vi "MHM ReadSens.vi"(8 "error in (no error)":errorcluster, 11 "ulMHMHandle":u32) -> (0 "error out":errorcluster, 2 "pSensorDataStruct":T1, 3 "function return":u32)   [LabVIEW 2019, in "MHM_1SL_interface.lvlib"]
uses:
  MHM_1SL_interface.lvlib
  lib/MHM_1SL_interface.dll
panel:
  in  "pSensorDataStruct":T1
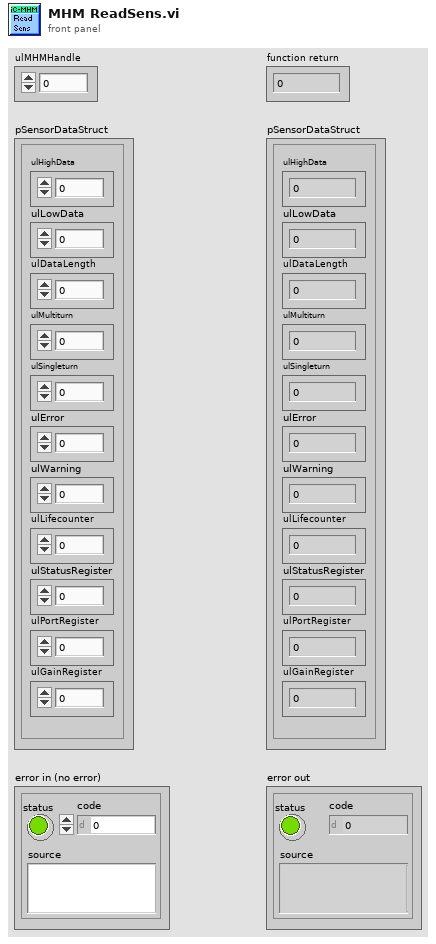
[diagram p1: front panel]
types:
  T1 = cluster{"ulHighData":u32, "ulLowData":u32, "ulDataLength":u32, "ulMultiturn":u32, "ulSingleturn":u32, "ulError":u32, "ulWarning":u32, "ulLifecounter":u32, "ulStatusRegister":u32, "ulPortRegister":u32, "ulGainRegister":u32}
  T2 = cluster{"pulMultiturn":u32, "pulSingleturn":u32, "pulError":u32, "pulWarning":u32, "pulLifecounter":u32, "pulStatusRegister":u32, "pulPortRegister":u32, "pulGainRegister":u32, "pulHighData":u32, "pulLowData":u32, "pulDataLength":u32}
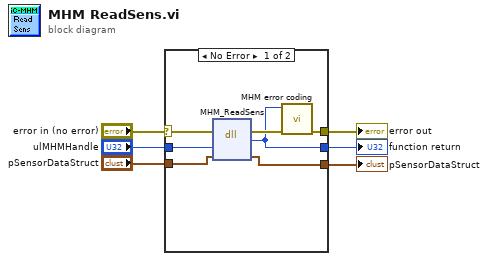
[diagram p0: block diagram]
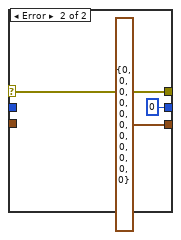
[diagram p2: hidden frame]
diagram:
  n1 = case shown="No Error" "error in (no error)" {
    selector: "error in (no error)" -> [w13 w16]
    tunnel: "ulMHMHandle" -> [w12 _]
    tunnel: [w10 w16] -> w4
    tunnel: [w9 u32 0 ("return type")] -> w3
    tunnel: "pSensorDataStruct" -> [w8 _]
    tunnel: [w7 T2 {"pulMultiturn"=0, "pulSingleturn"=0, "pulError"=0, "pulWarning"=0, "pulLifecounter"=0, "pulStatusRegister"=0, "pulPortRegister"=0, "pulGainRegister"=0, "pulHighData"=0, "pulLowData"=0, "pulDataLength"=0} ("pSensorDataStruct")] -> w1
    frame No Error {
      n2 = dll-call lib="C:/workspace/project/scancon/MHM_1SL_interface_4.4.0/lv_interface/lib/MHM_1SL_interface.dll" fn="MHM_ReadSens"(error in=w13, "ulMHMHandle"=w12, "pSensorDataStruct"=w8) -> (error out=w11:errorcluster, "return type"=w9:u32, "pSensorDataStruct"=w7:T1)  [unwired: 3 in, 1 out]
      n3 = call "MHM error coding.vi"("error in (no error)"=w11, "function return in"=w9) -> ("error out"=w10:errorcluster)  [unwired: 9 in]
    }
    frame Error {
    }
  }
  "function return" <- w3
  "error out" <- w4
  "pSensorDataStruct" <- w1
